vi "Read Table.vi"(0 "PDF Table Class.lvclass in":refnum<class "Pdfp Table Class.lvclass">, 7 "Row  [ ]":T7, 11 "error in (no error)":errorcluster) -> (2 "Table type":T20, 3 "Table columnWidth [ ]":sgl[](array[numeric]), 4 "PDF Table Class.lvclass out":refnum<class "Pdfp Table Class.lvclass">, 6 "Repeat on each new page?":bool, 8 "Image to Add [ ]":T21 {"Scale" format="%#_g %"}, 10 "Row format with ref [ ]":T6(array[cluster]), 13 "Titles and Datas 2D [ ]":string[][](array[string]), 14 "HeaderRows":u16, 15 "error out":errorcluster)   [LabVIEW 2019, in "Exaprom PDF.lvlib" / "Pdfp Table Class.lvclass"]
uses:
  Pdfp Table Class.lvclass
  Controls/General Controls/Image to Add [ ].ctl
  Controls/Image Controls/Image Scale.ctl
  Controls/Table Controls/Table type.ctl
  Controls/Table Controls/Table Appearance and Font Row [ ].ctl
  Controls/Table Controls/One Row Appearance.ctl
  Controls/Table Controls/Row from to.ctl
  Controls/Table Controls/Cell, Alignment, LS and Font - hide Vmerge.ctl
  Controls/Table Controls/Cell Type, Alignment and LS.ctl
  Controls/Table Controls/Cell Alignment 20px.ctl
  Controls/Table Controls/Text vertical arrangement.ctl
  Controls/Text Controls/Line spacing.ctl
  Controls/Table Controls/Cell Appearance.ctl
  Controls/Table Controls/Cell Border 20 px.ctl
  Controls/Table Controls/Merge Horizontal.ctl
  Controls/Table Controls/Merge Vertical.ctl
  Controls/Font Controls/Font complete cluster.ctl
  Controls/Font Controls/Font size.ctl
  Controls/Font Controls/Font color.ctl
  Controls/Font Controls/Type and encoding.ctl
  Controls/Text Controls/Unicode/Type and run direction.ctl
  Controls/Table Controls/Cell Cluster.ctl
  C:/work/niobrara_lv/labview pdf writer fixing/DLL/itextsharp.dll
  DLL/itextsharp.dll
  PDF Report Class/PDF Report Class.lvclass
  Pdfp Table Class.lvclass/Pdfp Table Class.ctl
  Exaprom PDF.lvlib
  Fonts Class/Font Class.lvclass
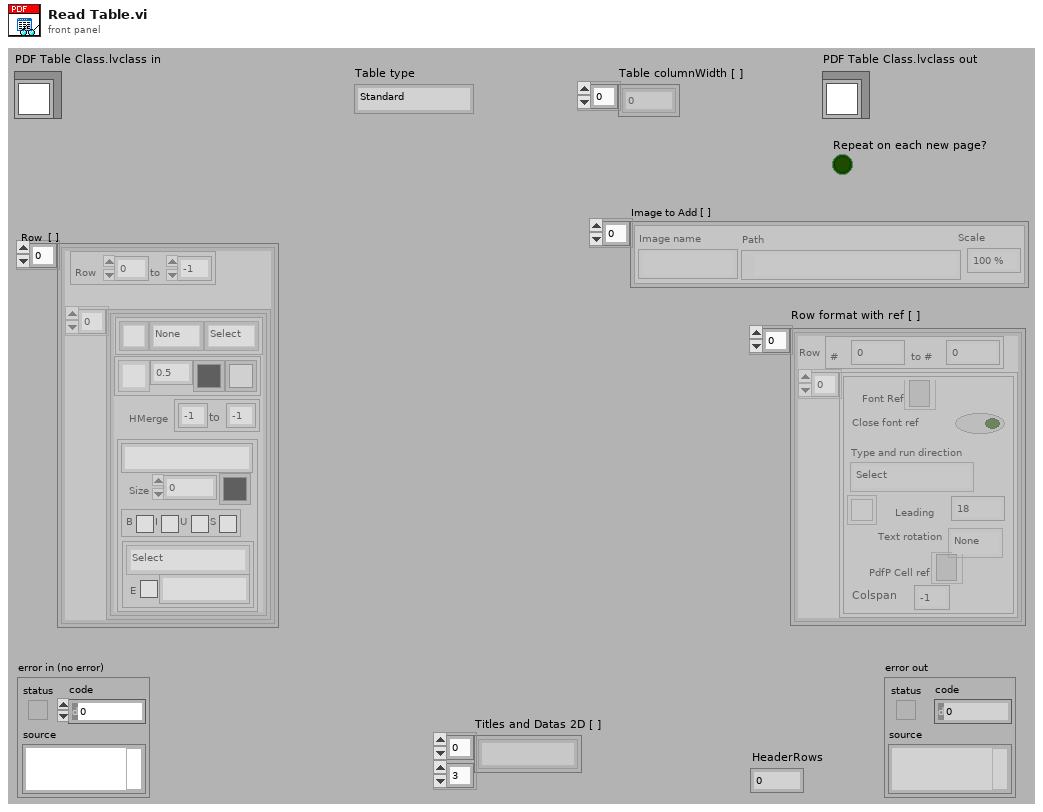
[diagram p1: front panel]
types:
  T1 = typedef "Exaprom PDF.lvlib/Cell Cluster.ctl" = cluster{"Font Ref":refnum<k24>, "Close font ref":bool, "Type and run direction":T2, "Cell Alignment":T3, "Text rotation":T4, "Leading":T5, "PdfP Cell ref":refnum<k24>, "Colspan":i8}
  T2 = typedef "Exaprom PDF.lvlib/Type and run direction.ctl" = enum16{"Select", "ASCII", "UTF-16", "UTF-16 (default)", "UTF-16 (LTR)", "UTF-16 (RTL)"}
  T3 = typedef "Exaprom PDF.lvlib/Cell Alignment 20px.ctl" = u16
  T4 = typedef "Exaprom PDF.lvlib/Text vertical arrangement.ctl" = enum16{"None", "Clockwise", "Counterclockwise"}
  T5 = typedef "Exaprom PDF.lvlib/Font size.ctl" = sgl
  T6 = cluster{"Row":cluster{"#":i16, "to #":i16}, "Cell [ ]":T1[]}[]
  T7 = typedef "Exaprom PDF.lvlib/Table Appearance and Font Row [ ].ctl" = T8[]
  T8 = typedef "Exaprom PDF.lvlib/One Row Appearance.ctl" = cluster{"Row":T9, "Cell [ ]":T10[]}
  T9 = typedef "Exaprom PDF.lvlib/Row from to.ctl" = cluster{"From #":i16, "to #":i16}
  T10 = typedef "Exaprom PDF.lvlib/Cell, Alignment, LS and Font - hide Vmerge.ctl" = cluster{"Text":T11, "Cell Appearance":T13, "HMerge":T15, "VMerge":T16, "Font":T17}
  T11 = typedef "Exaprom PDF.lvlib/Cell Type, Alignment and LS.ctl" = cluster{"Cell Alignment":T3, "Text rotation":T4, "Line spacing":T12}
  T12 = typedef "Exaprom PDF.lvlib/Line spacing.ctl" = enum16{"Select", "1.0", "1.5", "2.0"}
  T13 = typedef "Exaprom PDF.lvlib/Cell Appearance.ctl" = cluster{"Border":T14, "Thickness":sgl, "Color":u32, "BG":u32}
  T14 = typedef "Exaprom PDF.lvlib/Cell Border 20 px.ctl" = u16
  T15 = typedef "Exaprom PDF.lvlib/Merge Horizontal.ctl" = cluster{"From":i8, "to":i8}
  T16 = typedef "Exaprom PDF.lvlib/Merge Vertical.ctl" = cluster{"From":i8, "to":i8}
  T17 = typedef "Exaprom PDF.lvlib/Font complete cluster.ctl" = cluster{"Name":string, "Size":T5, "Color":T18, "Style":cluster{"Bold":bool, "Italic":bool, "Underline":bool, "Strikeout":bool}, "Type":T19}
  T18 = typedef "Exaprom PDF.lvlib/Font color.ctl" = u32
  T19 = typedef "Exaprom PDF.lvlib/Type and encoding.ctl" = cluster{"Type&direction":T2, "Embedded":bool, "Encoding":string}
  T20 = typedef "Exaprom PDF.lvlib/Table type.ctl" = enum16{"Standard", "Customized"}
  T21 = typedef "Exaprom PDF.lvlib/Image to Add [ ].ctl" = cluster{"Image name":string, "Path":path, "Scale":T22}[]
  T22 = typedef "Exaprom PDF.lvlib/Image Scale.ctl" = sgl
  T23 = typedef "Exaprom PDF.lvlib/System Fonts.ctl" = cluster{"Font name [ ]":string[], "Font and file names [ ]":cluster{"Font name":string, "File name":string}[]}
  T24 = typedef "Exaprom PDF.lvlib/Defaut Paragraphe and Line Spacing.ctl" = cluster{" Aligment":T25, "Line spacing":T12}
  T25 = typedef "Exaprom PDF.lvlib/Texte alignement.ctl" = enum16{"Select", "CENTER", "JUSTIFY", "LEFT", "RIGHT"}
  T26 = cluster{"Row":cluster{"#":i16, "to #":i16}, "Cell [ ]":T1[]}
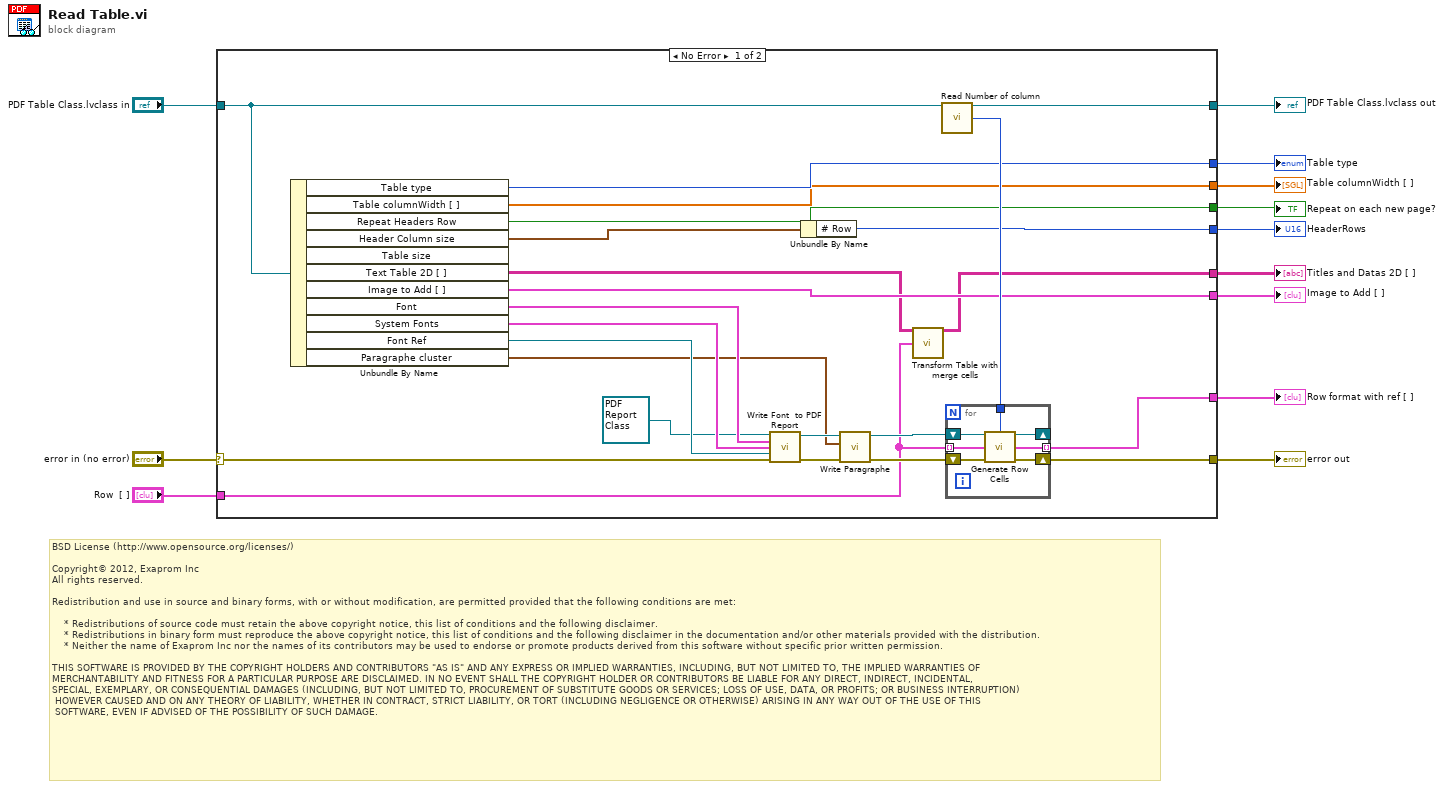
[diagram p0: block diagram]
diagram:
  # "BSD License (http://www.opensource.org/licenses/)\n\nCopyright© 2012, Exaprom Inc\nAll rights reserved.\n\nRedistribution and use in source and binary forms, with or without modification, are permitted provided that the following conditions are met:\n\n    * Redistributions of source code must retain the above copyright notice, this list of conditions and the following disclaimer.\n    * Redistributions in binary form must reproduce the above copyright notice, this list of conditions and the following disclaimer in the documentation and/or other materials provided with the distribution.\n    * Neither the name of Exaprom Inc nor the names of its contributors may be used to endorse or promote products derived from this software without specific prior written permission.\n\nTHIS SOFTWARE IS PROVIDED BY THE COPYRIGHT HOLDERS AND CONTRIBUTORS \"AS IS\" AND ANY EXPRESS OR IMPLIED WARRANTIES, INCLUDING, BUT NOT LIMITED TO, THE IMPLIED WARRANTIES OF \nMERCHANTABILITY AND FITNESS FOR A PARTICULAR PURPOSE ARE DISCLAIMED. IN NO EVENT SHALL THE COPYRIGHT HOLDER OR CONTRIBUTORS BE LIABLE FOR ANY DIRECT, INDIRECT, INCIDENTAL,\nSPECIAL, EXEMPLARY, OR CONSEQUENTIAL DAMAGES (INCLUDING, BUT NOT LIMITED TO, PROCUREMENT OF SUBSTITUTE GOODS OR SERVICES; LOSS OF USE, DATA, OR PROFITS; OR BUSINESS INTERRUPTION)\n HOWEVER CAUSED AND ON ANY THEORY OF LIABILITY, WHETHER IN CONTRACT, STRICT LIABILITY, OR TORT (INCLUDING NEGLIGENCE OR OTHERWISE) ARISING IN ANY WAY OUT OF THE USE OF THIS\n SOFTWARE, EVEN IF ADVISED OF THE POSSIBILITY OF SUCH DAMAGE."
  n1 = case shown="No Error" "error in (no error)" {
    selector: "error in (no error)" -> [w28 w44]
    tunnel: [w36 w44] -> w11
    tunnel: [w33 w45] -> w9
    tunnel: "PDF Table Class.lvclass in" -> [w34 w45]
    tunnel: [w19 _] -> w8
    tunnel: [w20 _] -> w7
    tunnel: [w35 _] -> w1
    tunnel: [w13 _] -> w6
    tunnel: [w16 _] -> w5
    tunnel: [w21 _] -> w4
    tunnel: [w17 _] -> w3
    tunnel: "Row  [ ]" -> [w14 _]
    frame No Error {
      n2 = Unbundle By Name(w34) -> ("Table type"=w21:T20, "Table columnWidth [ ]"=w20:sgl[], "Repeat Headers Row"=w19:bool, "Header Column size"=w18:cluster{"# Column":u16, "# Row":u16}, "Text Table 2D [ ]"=w15:string[][], "Image to Add [ ]"=w16:T21, "Font"=w31:T17, "System Fonts"=w30:T23, "Font Ref"=w29:refnum<k24>, "Paragraphe cluster"=w23:T24)  [unwired: 1 out]
      n3 = call "Write Font  to PDF Report.vi"("PDF Report IN"=refnum<class "PDF Report Class.lvclass"> refnum, "Font"=w31, "System Fonts"=w30, "Font Ref"=w29, "error in (no error)"=w28) -> ("PDF Report OUT"=w24:refnum<class "PDF Report Class.lvclass">, "error out"=w27:errorcluster)  [unwired: 9 in]
      n4 = Unbundle By Name(w18) -> ("# Row"=w17:u16)
      n5 = call-dynamic "Write Paragraphe.vi"("error in (no error)"=w27, "Paragraphe cluster"=w23, "PDF Report Class in"=w24) -> ("error out"=w25:errorcluster, "PDF Report Class out"=w22:refnum<class "PDF Report Class.lvclass">)  [unwired: 7 in]
      n6 = call "Transform Table with merge cells.vi"("Titles and Datas 2D [ ] IN"=w15, "Row  [ ]"=w14) -> ("Titles and Datas 2D [ ] OUT"=w13:string[][])  [unwired: 12 in, 1 out]
      n7 = call "Read Number of column.vi"("PDF Table Class"=w34) -> ("PDF Table Class duplicate"=w33:refnum<class "Pdfp Table Class.lvclass">, "# columns"=w32:i32)  [unwired: 1 in, 12 out]
      n8 = for "Number of titles rows" {
        tunnel: w14 -> [w37] mode=indexing
        shift-right: [w43] -> w36
        shift-left: w25 -> [w42]
        shift-right: [w41] -> _
        shift-left: w22 -> [w40]
        tunnel: [w39] -> w35 mode=indexing
        tunnel: w32 -> [w38]
        n9 = call "Generate Row Cells.vi"("PDF Report"=w40, "Number Colum"=w38, "Row Borders"=w37, "error in (no error)"=w42) -> ("PDF Report duplicate"=w41:refnum<class "PDF Report Class.lvclass">, "Row format with ref"=w39:T26, "error out"=w43:errorcluster)  [unwired: 9 out]
      }
    }
    frame Error {
    }
  }
  "error out" <- w11
  "PDF Table Class.lvclass out" <- w9
  "Repeat on each new page?" <- w8
  "Table columnWidth [ ]" <- w7
  "HeaderRows" <- w3
  "Titles and Datas 2D [ ]" <- w6
  "Image to Add [ ]" <- w5
  "Table type" <- w4
  "Row format with ref [ ]" <- w1
